vi "PH_PPMA_PowerUnit.src PSU.vi"(0 "i ref in":refnum<vi>, 5 "error in (no error)":errorcluster) -> (14 "i ref out":refnum<vi>, 19 "error out":errorcluster)   [LabVIEW 2014, in "PH_PPMA_PowerUnit.lvlib"]
doc: "This is the action VI of the _StatePSU event case. If \n\n1: if SM State = \"Switch PSU off\", a state change request is send to SM to get \"Open Ross Relais\"\n\nIt finally calls \"State PU\""
uses:
  PH_PPMA_PowerUnit.lvlib
  PH_Basics/PH_PowerUnit_BaseClass/PH_PowerUnit_BaseClass.SM States.ctl
  PH_Basics/PH_PowerUnit_BaseClass/PH_PowerUnit_BaseClass.lvlib
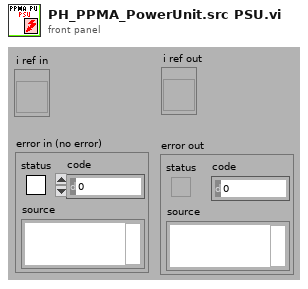
[diagram p1: front panel]
types:
  T1 = typedef "PH_PPMA_PowerUnit.lvlib/PH_PPMA_PowerUnit.i attribute.ctl" = cluster{"GUI Refs":cluster{"Rods":refnum<vi>, "Ignitron":refnum<vi>, "Rossrelais":refnum<vi>, "Set Voltage":refnum<vi>, "PSU":refnum<vi>, "EOC":refnum<vi>, "Trigger":refnum<vi>}, "Rods":T2, "PSU":T4, "Ross Relais":T5, "Ignitron":T6, "Trigger":cluster{"State Device":T3, "linked?":bool}, "Timing Settings":cluster{"Prdc Fast?":bool, "Default Value Periodic Interval":i32, "Mercury on since":dbl, "Warm up Time Mercury [s]":dbl}, "Set Voltage [V]":dbl}
  T2 = typedef "PH_PPMA_PowerUnit.lvlib/PH_PPMA_PowerUnit.Rods Attributes.ctl" = cluster{"Instancename":string, "Device Status":T3, "linked?":bool}
  T3 = typedef "PH_StatusHandler.lvlib/PH_StatusHandler.Status.ctl" = i16
  T4 = typedef "PH_PP_Common.lvlib/PH_PP_Common.PSU Attributes.ctl" = cluster{"lower limit [V]":dbl, "upper limit [V]":dbl, "Voltage set":bool, "State Device":T3, "linked?":bool}
  T5 = typedef "PH_PP_Common.lvlib/PH_PP_Common.Ross Relais Attributes.ctl" = cluster{"State Device":T3, "linked?":bool}
  T6 = typedef "PH_PP_Common.lvlib/PH_PP_Common.Ignitron Attributes.ctl" = cluster{"State Device":T3, "linked?":bool}
  T7 = typedef "PH_PowerUnit_BaseClass.lvlib/PH_PowerUnit_BaseClass.SM States.ctl" = enum16{".", "Stand by", "Switch PU on", "Configure", "Set Default Voltage", "Set STANDBY", "Set READY", "Wait for Shot Cmd", "Open Dump Rods", "Open Ross Relais", "Close Ross Relais", "Switch PSU on", "Switch PSU off", "Charge", "Switch GD Channel on", "Close Dump Rods", "Rods-TO", "RR-TO", "PSU-TO", "Trigger-TO"}
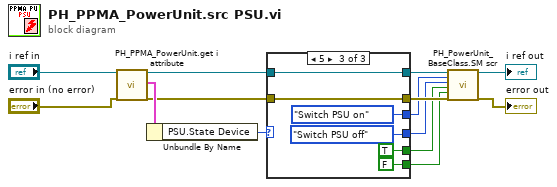
[diagram p0: block diagram]
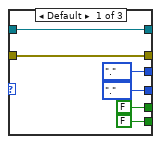
[diagram p2: hidden frame]
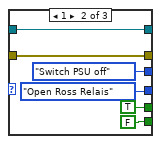
[diagram p3: hidden frame]
diagram:
  n1 = call "PH_PPMA_PowerUnit.get i attribute.vi"("i ref in"="i ref in", "error in (no error)"="error in (no error)") -> ("i ref out"=w11:refnum<vi>, "i attribute"=w14:T1, "error out"=w10:errorcluster)  [unwired: 15 in]
  n2 = Unbundle By Name(w14) -> ("PSU.State Device"=w9:T3)
  n3 = case shown="5" w9 {
    tunnel: w11 -> [w20 w22 w28]
    tunnel: w10 -> [w19 w21 w27]
    tunnel: [w19 w21 w27] -> w8
    tunnel: [w20 w22 w28] -> w6
    tunnel: [PH_PowerUnit_BaseClass.SM_States."." ("Current SM State (condition)") PH_PowerUnit_BaseClass.SM_States."Switch PSU off" ("Current SM State (condition)") PH_PowerUnit_BaseClass.SM_States."Switch PSU on" ("Current SM State (condition)")] -> w4
    tunnel: [PH_PowerUnit_BaseClass.SM_States."." ("Current SM State (condition)") PH_PowerUnit_BaseClass.SM_States."Open Ross Relais" ("Current SM State (condition)") PH_PowerUnit_BaseClass.SM_States."Switch PSU off" ("Current SM State (condition)")] -> w3
    tunnel: [FALSE TRUE TRUE] -> w2
    tunnel: [FALSE FALSE FALSE] -> w1
    frame Default {
    }
    frame 1 {
    }
    frame 5 {
    }
  }
  n4 = call "PH_PowerUnit_BaseClass.SM scr.vi"("VI in"=w6, "Current SM State (condition)"=w4, "Wanted SM State"=w3, "Further change condition"=w2, "PU in use is condition? (true)"=w1, "error in (no error)"=w8) -> ("VI out"=→"i ref out":refnum<vi>, "error out"=→"error out":errorcluster)  [unwired: 12 in]
